vi "Thermistor, SP21629.vi"(8 "error in":errorcluster, 11 "resistance (ohms)":dbl=59082.262 format="%.3f") -> (0 "error out":errorcluster, 3 "temperature (C)":dbl=nan format="%.3f")   [LabVIEW 2020]
doc: "This function converts an SP21629 thermistor resistance (ohms) to temperature (Celsius) using a spline interpolation of the specifications in the manufacturer's datasheet."
uses:
  <vilib>/gmath/NI_Gmath.lvlib
panel:
  in  "Excel Clipboard to Import (SP21629 Datasheet)":string="0.0\t351017.0\n1.0\t332620.0\n2.0\t315288.0\n3.0\t298954.0\n4.0\t283555.0\n5.0\t269034.0\n6.0\t255335.0\n7.0\t242408.0\n8.0\t230206.0\n9.0\t218684.0\n10.0\t207801.0\n11.0\t197518.0\n12.0\t187799.0\n13.0\t178610.0\n14.0\t169921.0\n15.0\t161700.0\n16.0\t153921.0\n17.0\t146558.0\n18.0\t139586.0\n19.0\t132983.0\n20.0\t126727.0\n21.0\t120799.0\n22.0\t115179.0\n23.0\t109850.0\n24.0\t104795.0\n25.0\t100000.0\n26.0\t95449.0\n27.0\t91129.0\n28.0\t87027.0\n29.0\t83131.0\n30.0\t79430.0\n31.0\t75913.0\n32.0\t72569.0\n33.0\t69390.0\n34.0\t66367.0\n35.0\t63491.0\n36.0\t60755.0\n37.0\t58150.0\n38.0\t55670.0\n39.0\t53309.0\n40.0\t51060.0\n41.0\t48917.0\n42.0\t46875.0\n43.0\t44929.0\n44.0\t43073.0\n45.0\t41303.0\n46.0\t39615.0\n47.0\t38005.0\n48.0\t36467.0\n49.0\t35000.0\n50.0\t33599.0\n51.0\t32262.0\n52.0\t30984.0\n53.0\t29763.0\n54.0\t28596.0\n55.0\t27481.0\n56.0\t26415.0\n57.0\t25395.0\n58.0\t24420.0\n59.0\t23487.0\n60.0\t22594.0\n61.0\t21740.0\n62.0\t20922.0\n63.0\t20138.0\n64.0\t19388.0\n65.0\t18670.0\n66.0\t17981.0\n67.0\t17322.0\n68.0\t16689.0\n69.0\t16083.0\n70.0\t15502.0\n"
  in  "SP21629 Specifications (0 to 70 C)":string[][](table)=[["0.0", "351017.0"], ["1.0", "332620.0"], ["2.0", "315288.0"], ["3.0", "298954.0"], ["4.0", "283555.0"], ["5.0", "269034.0"], ["6.0", "255335.0"], ["7.0", "242408.0"], ["8.0", "230206.0"], ["9.0", "218684.0"], ["10.0", "207801.0"], ["11.0", "197518.0"], ["12.0", "187799.0"], ["13.0", "178610.0"], ["14.0", "169921.0"], ["15.0", "161700.0"], ["16.0", "153921.0"], ["17.0", "146558.0"], ["18.0", "139586.0"], ["19.0", "132983.0"], ["20.0", "126727.0"], ["21.0", "120799.0"], ["22.0", "115179.0"], ["23.0", "109850.0"], ["24.0", "104795.0"], ["25.0", "100000.0"], ["26.0", "95449.0"], ["27.0", "91129.0"], ["28.0", "87027.0"], ["29.0", "83131.0"], ["30.0", "79430.0"], ["31.0", "75913.0"], ["32.0", "72569.0"], ["33.0", "69390.0"], ["34.0", "66367.0"], ["35.0", "63491.0"], ["36.0", "60755.0"], ["37.0", "58150.0"], ["38.0", "55670.0"], ["39.0", "53309.0"], ["40.0", "51060.0"], ["41.0", "48917.0"], ["42.0", "46875.0"], ["43.0", "44929.0"], ["44.0", "43073.0"], ["45.0", "41303.0"], ["46.0", "39615.0"], ["47.0", "38005.0"], ["48.0", "36467.0"], ["49.0", "35000.0"], ["50.0", "33599.0"], ["51.0", "32262.0"], ["52.0", "30984.0"], ["53.0", "29763.0"], ["54.0", "28596.0"], ["55.0", "27481.0"], ["56.0", "26415.0"], ["57.0", "25395.0"], ["58.0", "24420.0"], ["59.0", "23487.0"], ["60.0", "22594.0"], ["61.0", "21740.0"], ["62.0", "20922.0"], ["63.0", "20138.0"], ["64.0", "19388.0"], ["65.0", "18670.0"], ["66.0", "17981.0"], ["67.0", "17322.0"], ["68.0", "16689.0"], ["69.0", "16083.0"], ["70.0", "15502.0"]]
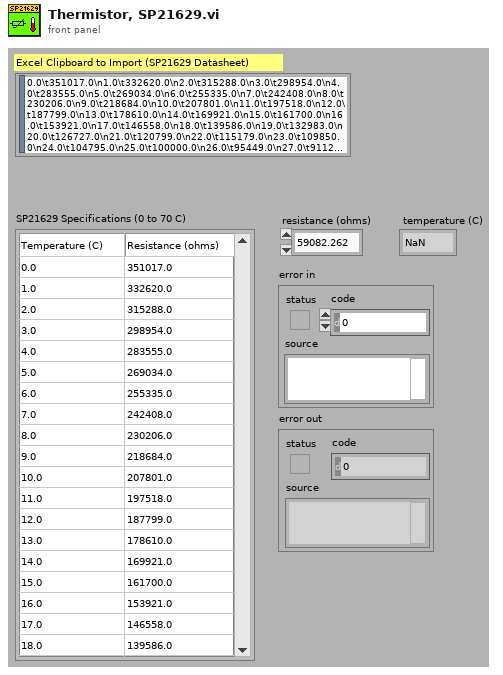
[diagram p1: front panel]
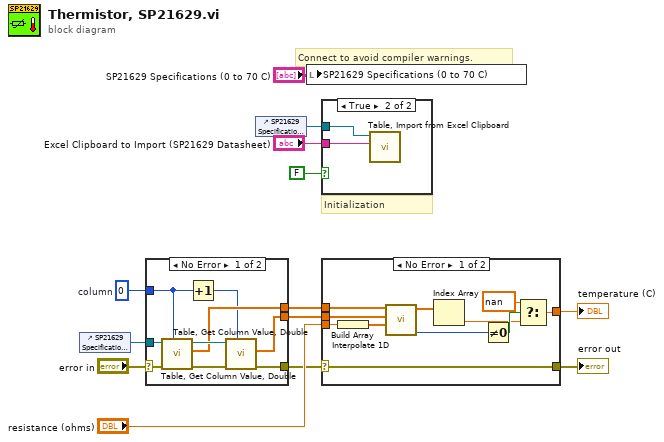
[diagram p0: block diagram]
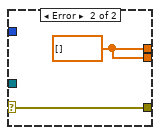
[diagram p2: hidden frame]
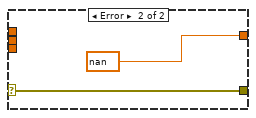
[diagram p3: hidden frame]
diagram:
  w4 = 0  # column
  # "Connect to avoid compiler warnings."
  # "Initialization"
  n1 = control-ref of="SP21629 Specifications (0 to 70 C)"() -> (w10:refnum<vi>)
  n2 = case shown="No Error" "error in" {
    selector: "error in" -> [w14 w24]
    tunnel: w10 -> [w22 _]
    tunnel: [w19 w23] -> w8
    tunnel: [w18 w23] -> w7
    tunnel: w4 -> [w17 _]
    tunnel: [w15 w24] -> w3
    frame No Error {
      n3 = call "Table, Get Column Value, Double.vi"("error in"=w14, "Tbl Refnum"=w22, "column (0)"=w17) -> ("error out"=w20:errorcluster, "Value"=w19:dbl[], "Tbl Refnum out"=w21:refnum<vi>)  [unwired: 5 in]
      n4 = Increment(x=w17) -> (x+1=w16:i32)
      n5 = call "Table, Get Column Value, Double.vi"("error in"=w20, "Tbl Refnum"=w21, "column (0)"=w16) -> ("error out"=w15:errorcluster, "Value"=w18:dbl[])  [unwired: 5 in, 1 out]
    }
    frame Error {
      w23 = dbl[] [] ("Value")
    }
  }
  n6 = control-ref of="SP21629 Specifications (0 to 70 C)"() -> (w12:refnum<vi>)
  n7 = local write "SP21629 Specifications (0 to 70 C)"("SP21629 Specifications (0 to 70 C)") -> ()
  n8 = case shown="True" FALSE {
    tunnel: "Excel Clipboard to Import (SP21629 Datasheet)" -> [_ w26]
    tunnel: w12 -> [_ w25]
    frame False {
    }
    frame True {
      n9 = call "Table, Import from Excel Clipboard.vi"("Excel Clipboard to Import"=w26, "Tbl Refnum"=w25) -> ()  [unwired: 8 in, 2 out]
    }
  }
  n10 = case shown="No Error" w3 {
    selector: w3 -> [w32 w38]
    tunnel: w8 -> [w37 _]
    tunnel: w7 -> [w36 _]
    tunnel: [w30 nan ("Numeric")] -> w6
    tunnel: "resistance (ohms)" -> [w33 _]
    tunnel: [w32 w38] -> w2
    frame No Error {
      n11 = Build Array(w33) -> (w34:dbl[])
      n12 = call <vilib>:"Interpolate 1D.vi"("xi"=w34, "X"=w36, "Y"=w37) -> ("error"=w31:i32, "yi"=w35:dbl[])  [unwired: 6 in, 1 out]
      n13 = Index Array(array=w35) -> (element=w28:dbl)  [unwired: 1 in]
      n14 = Not Equal To 0?(x=w31) -> (x != 0?=w29:bool)
      n15 = Select(t=nan, s=w29, f=w28) -> (s? t:f=w30:dbl)
    }
    frame Error {
    }
  }
  "temperature (C)" <- w6
  "error out" <- w2
